vi "Match value to sensitivity.vi"(11 "integer":i8) -> (3 "sensitivity":dbl[unit])   [LabVIEW 2017, in "SR830.lvlib"]
doc: "Takes an integer input (the value returned by the lock-in) and matches it to its corresponding time constant."
uses:
  SR830.lvlib
  time constants.ctl
panel:
  in  "Lock-in sensitivity settings (ring)\n(in nanovolts)":T1 items=["0"=2.0, "1"=5.0, "2"=10.0, "3"=20.0, "4"=50.0, "5"=100.0, "6"=200.0, "7"=500.0, "8"=1000.0, "9"=2000.0, "10"=5000.0, "11"=10000.0, "12"=20000.0, "13"=50000.0, "14"=100000.0, "15"=200000.0, "16"=500000.0, "17"=1000000.0, "18"=2000000.0, "19"=5000000.0, "20"=10000000.0, "21"=20000000.0, "22"=50000000.0, "23"=100000000.0, "24"=200000000.0, "25"=500000000.0, "26"=1000000000.0]
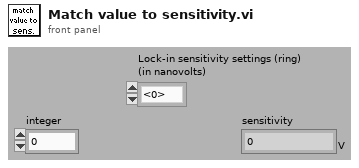
[diagram p1: front panel]
types:
  T1 = typedef "SR830.lvlib/time constants.ctl" = dbl
  T2 = typedef "LVStringsAndValuesArrayTypeDef_DBL.ctl" = cluster{"String":string, "Value":dbl}[]
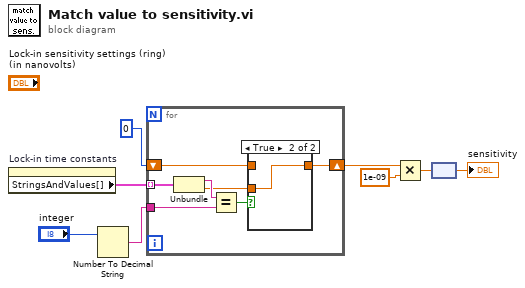
[diagram p0: block diagram]
diagram:
  n1 = property on="Lock-in time constants" class="Ring (strict)"() -> ("StringsAndValues[]"=w5:T2)  [unwired: 2 in, 2 out]
  n2 = Number To Decimal String(number="integer") -> (decimal integer string=w7:string)  [unwired: 1 out]
  n3 = for {
    tunnel: w5 -> [w11] mode=indexing
    tunnel: w7 -> [w15]
    shift-right: [w13] -> w3
    shift-left: 0 -> [w12]
    n4 = Unbundle(w11) -> ("String"=w10:string, "Value"=w9:dbl)
    n5 = Equal?(x=w10, y=w15) -> (x = y?=w14:bool)
    n6 = case shown="True" w14 {
      tunnel: [w16 w17] -> w13
      tunnel: w12 -> [w16 _]
      tunnel: w9 -> [_ w17]
      frame False {
      }
      frame True {
      }
    }
  }
  n7 = Multiply(x=w3, y=1e-09) -> (x*y=w2:dbl)
  n8 = node(w2) -> (→"sensitivity":dbl[unit])
